vi "Initialise.vi"(11 "Diffuse Colour":refnum<vi>) -> (3 "Core Data out":T1)   [LabVIEW 2020, in "Example 1.lvlib"]
uses:
  Example 1.lvlib
  Graphics/Libraries/Raster/Rectangle Dimensions.ctl
  Graphics/Libraries/Raster/Raster.lvlib
  Core Data.ctl
  Scene/Scene.lvclass
  Scene/Mouse Button Held.ctl
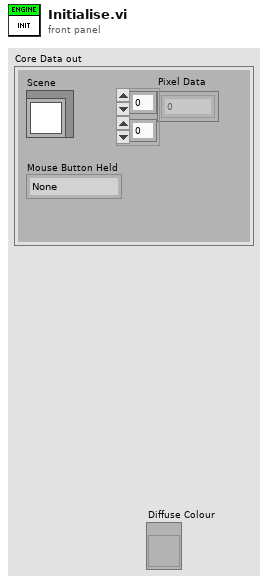
[diagram p1: front panel]
types:
  T1 = typedef "Example 1.lvlib/Core Data.ctl" = cluster{"Pixel Data":u32[][], "Scene":refnum<class "Scene.lvclass">, "Mouse Button Held":T2}
  T2 = typedef "Scene.lvclass/Mouse Button Held.ctl" = enum16{"None", "Left", "Middle", "Right"}
  T3 = typedef "Raster.lvlib/Rectangle Dimensions.ctl" = cluster{"Width":u32, "Height":u32}
  T4 = enum32{"invalid app kind", "Development System", "Run Time System", "Student Edition", "Embedded LabVIEW", "Evaluation", "Custom"}
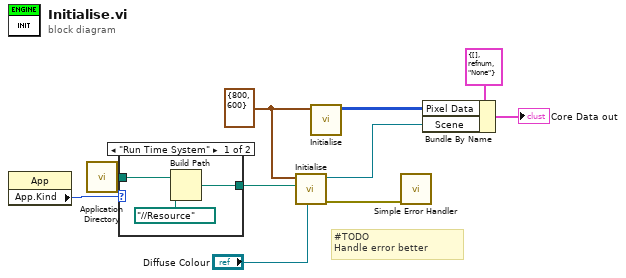
[diagram p0: block diagram]
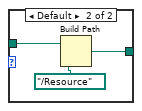
[diagram p2: hidden frame]
diagram:
  w3 = T3 {"Width"=800, "Height"=600} ("Screen Dimensions")
  # "#TODO\nHandle error better"
  n1 = property class="App"() -> ("App.Kind"=w6:T4)  [unwired: 2 in, 2 out]
  n2 = call <vilib>:"Application Directory.vi"() -> ("Application Directory"=w4:path)
  n3 = case shown="\"Run Time System\"" w6 {
    tunnel: [w13 w16] -> w5
    tunnel: w4 -> [w11 w14]
    frame "Run Time System" {
      n4 = Build Path(base path=w11, name or relative path=path "../../Resource") -> (appended path=w13:path)
    }
    frame Default {
      n5 = Build Path(base path=w14, name or relative path=path "../Resource") -> (appended path=w16:path)
    }
  }
  n6 = call "Initialise.vi"("Diffuse Colour"="Diffuse Colour", "Resource Directory"=w5, "Screen Dimensions"=w3) -> ("error out"=w7:errorcluster, "Scene out"=w1:refnum<class "Scene.lvclass">)  [unwired: 7 in]
  n7 = call "Initialise.vi"("Screen Dimensions"=w3) -> ("Pixel Data out"=w8:u32[][])  [unwired: 10 in]
  n8 = call <vilib>:"Simple Error Handler.vi"("error in (no error)"=w7) -> ()  [unwired: 4 in, 5 out]
  n9 = Bundle By Name(cluster=T1 {"Pixel Data"=[], "Scene"=refnum, "Mouse Button Held"=enum."None"} ("Core Data"), "Pixel Data"=w8, "Scene"=w1) -> (→"Core Data out":T1)
